vi "range_filter.vi"(0 "array input":dbl[](array[numeric]), 2 "upper limit":dbl=1.0 format="%#_13g", 3 "lower limit":dbl=-1.0 format="%#_13g") -> (8 "Array output":dbl[](array[numeric]))   [LabVIEW 2020]
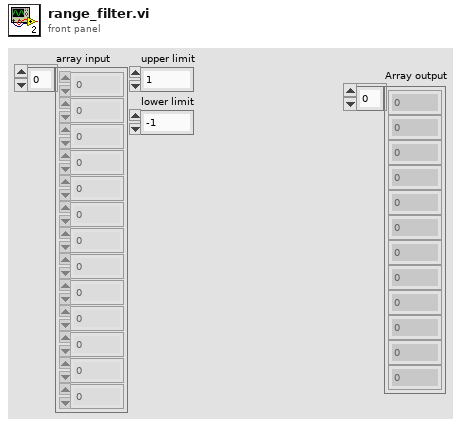
[diagram p1: front panel]
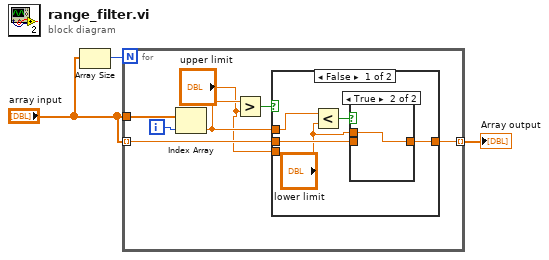
[diagram p0: block diagram]
diagram:
  n1 = Array Size(array="array input") -> (size(s)=w3:i32)
  n2 = for {
    N: w3 -> [_]
    tunnel: "array input" -> [w9]
    tunnel: [w6] -> w2 mode=indexing
    tunnel: "array input" -> [w5] mode=indexing
    i -> [w10]
    n3 = Index Array(array=w9, index=w10) -> (element=w7:dbl)
    n4 = Greater?(x=w7, y="upper limit") -> (0:w8:bool)
    n5 = case shown="False" w8 {
      tunnel: w7 -> [w15 _]
      tunnel: [w13 w18] -> w6
      tunnel: w5 -> [w12 _]
      tunnel: "upper limit" -> [_ w18]
      frame False {
        n6 = Less?(x=w15, y="lower limit") -> (x < y?=w14:bool)
        n7 = case shown="True" w14 {
          tunnel: [w16 w17] -> w13
          tunnel: w12 -> [w16 _]
          tunnel: "lower limit" -> [_ w17]
          frame False {
          }
          frame True {
          }
        }
      }
      frame True {
      }
    }
  }
  "Array output" <- w2
